vi "TestLibGetFileTime.vi"() -> ()   [LabVIEW 2020]
uses:
  LabviewTools32.dll
panel:
  out "Array 2":i32[](array[numeric])
  out "Array":T1(array[cluster])
  in  "Path":path=path "C:/Factory/FactoryProductTestTool/Sequences"
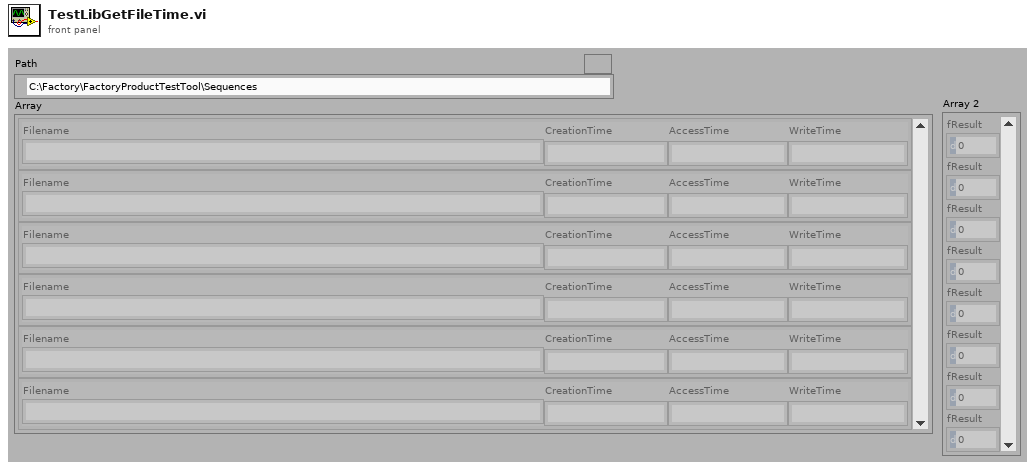
[diagram p1: front panel]
types:
  T1 = cluster{"Filename":string, "CreationTime":string, "AccessTime":string, "WriteTime":string}[]
  T2 = cluster{"Filename":string, "CreationTime":string, "AccessTime":string, "WriteTime":string}
  T3 = cluster{"wYear":u16, "wMonth":u16, "wDayOfWeek":u16, "wDay":u16, "wHour":u16, "wMinute":u16, "wSeconde":u16, "wMilliSeconds":u16}
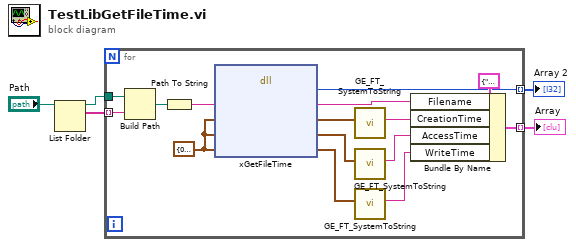
[diagram p0: block diagram]
diagram:
  n1 = List Folder(path="Path") -> (path out=w3:path, filenames=w4:string[])  [unwired: 3 in, 2 out]
  n2 = for {
    tunnel: w4 -> [w17] mode=indexing
    tunnel: w3 -> [w19]
    tunnel: [w15] -> w2 mode=indexing
    tunnel: [w6] -> w1 mode=indexing
    w14 = T3 {"wYear"=0, "wMonth"=0, "wDayOfWeek"=0, "wDay"=0, "wHour"=0, "wMinute"=0, "wSeconde"=0, "wMilliSeconds"=0} ("System")
    n3 = Build Path(base path=w19, name or relative path=w17) -> (appended path=w18:path)
    n4 = Path To String(path=w18) -> (string=w20:string)
    n5 = dll-call lib="C:/Factory/FactoryGenericTools/Dll/LabviewTools32.dll" fn="xGetFileTime"("cPath"=w20, "vCreationTime"=w14, "vAccessTime"=w14, "vWriteTime"=w14) -> ("fResult"=w6:i32, "cPath"=w16:string, "vCreationTime"=w12:T3, "vAccessTime"=w11:T3, "vWriteTime"=w8:T3)  [unwired: 3 in, 2 out]
    n6 = call "GE_FT_SystemToString.vi"("SystemTime"=w12) -> ("FileTimeString"=w10:string)  [unwired: 9 in, 1 out]
    n7 = call "GE_FT_SystemToString.vi"("SystemTime"=w11) -> ("FileTimeString"=w9:string)  [unwired: 9 in, 1 out]
    n8 = call "GE_FT_SystemToString.vi"("SystemTime"=w8) -> ("FileTimeString"=w7:string)  [unwired: 9 in, 1 out]
    n9 = Bundle By Name(cluster=T2 {"Filename"="", "CreationTime"="", "AccessTime"="", "WriteTime"=""}, "Filename"=w16, "CreationTime"=w10, "AccessTime"=w9, "WriteTime"=w7) -> (w15:T2)
  }
  "Array" <- w2
  "Array 2" <- w1
